vi "qnet_mechkit_decoder.vi"(1 "Reload Value":i16, 2 "Reset":bool, 3 "Z":bool, 4 "B":bool, 5 "A":bool, 6 "Enable Index":bool) -> (0 "16 bit Position":i16)   [LabVIEW 2017]
doc: "This contains a quadrature decoder with basic index support. When the index is enabled, the counter is reset to a specified value when the index pulse goes high or to zero if the reset button has been clicked."
uses:
  <vilib>/Simulation/Implementation/Shared/SIMSCR Execution Mode.ctl
  <vilib>/Simulation/Scripting/Companion Diagram/SimConfigNode/SimParams.ctl
  <vilib>/Simulation/Scripting/Companion Diagram/SimConfigNode/_simSolvers.ctl
  <vilib>/Simulation/Param Hierarchy/Typedefs/SIMPH Param Control Actions.ctl
  <vilib>/Simulation/Implementation/Shared/NILVSim_ParamChanged.vi
  <vilib>/Simulation/Implementation/Shared/NILVSIM_BeginStep.vi
  <vilib>/Simulation/Utility/Implementation/NILVSim Memory.llb/NILVSim Memory (core).vi
  <vilib>/Simulation/Implementation/Shared/NILVSim_Manager.vi
  <vilib>/Utility/error.llb/Clear Errors.vi
  <vilib>/Simulation/Implementation/Shared/NILVSim_FinalizeModel.vi
  <vilib>/Simulation/Implementation/Shared/SIM Unbundle Sim Info.vi
  <vilib>/Simulation/Implementation/Shared/SIMSH Read Queue.vi
  <vilib>/Simulation/Implementation/Shared/NILVSim_Initialize.vi
  <vilib>/Simulation/Utility/Implementation/NILVSim Get Time and IsAcceptedStep.vi
  <vilib>/Simulation/Implementation/Shared/NILVSim_GetModelError.vi
  <vilib>/Simulation/Implementation/Shared/SIM SimErrorHandler.vi
  <vilib>/Simulation/Implementation/Shared/SIM Bundle Sim Info.vi
  <vilib>/Simulation/Scripting/Companion Diagram/SimConfigNode/SimDog.xnode
  <vilib>/Simulation/Implementation/XNodeFramework/SimXNode/SimX.xnode
  <vilib>/Simulation/Implementation/Shared/NI_SIM_Implementation.lvlib
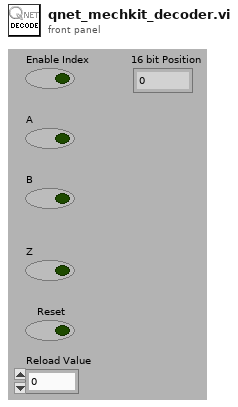
[diagram p1: front panel]
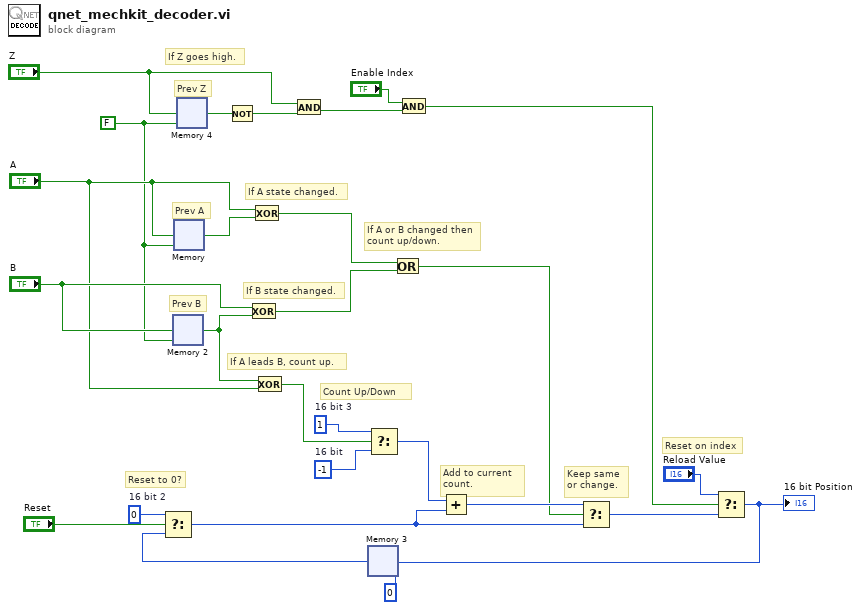
[diagram p0: block diagram]
diagram:
  w1 = FALSE ("initial value 2")
  w16 = i16 -1  # 16 bit
  w15 = i16 1  # 16 bit 3
  w11 = i16 0  # 16 bit 2
  # "Prev Z"
  # "If Z goes high."
  # "Add to current \ncount."
  # "Prev B"
  # "Prev A"
  # "Reset to 0?"
  # "Reset on index"
  # "Count Up/Down"
  # "Keep same \nor change."
  # "If A leads B, count up."
  # "If A state changed."
  # "If B state changed."
  # "If A or B changed then count up/down."
  n1 = xnode ("Memory 2")("input"="B", "initial value"=w1) -> ("output"=w20:bool)  [unwired: 4 in]
  n2 = xnode ("Memory")("input"="A", "initial value"=w1) -> ("output"=w19:bool)  [unwired: 4 in]
  n3 = xnode ("Memory 4")("input"="Z", "initial value"=w1) -> ("output"=w4:bool)  [unwired: 4 in]
  n4 = Not(x=w4) -> (.not. x?=w5:bool)
  n5 = Exclusive Or ("Exclusive Or 2")(1:w20, 2:"B") -> (0:w9:bool)
  n6 = Exclusive Or(1:w19, 2:"A") -> (0:w18:bool)
  n7 = Exclusive Or ("Exclusive Or 3")(1:"A", 2:w20) -> (0:w8:bool)
  n8 = And ("And 2")(x="Z", y=w5) -> (x .and. y?=w3:bool)
  n9 = Select ("Select 3")(t=w15, s=w8, f=w16) -> (s? t:f=w14:i16)
  n10 = Or(x=w18, y=w9) -> (x .or. y?=w7:bool)
  n11 = And(x="Enable Index", y=w3) -> (x .and. y?=w25:bool)
  n12 = Select ("Select 2")(t=w11, s="Reset", f=w21) -> (s? t:f=w12:i16)
  n13 = Add(x=w14, y=w12) -> (x+y=w10:i16)
  n14 = Select(t=w10, s=w7, f=w12) -> (s? t:f=w17:i16)
  n15 = Select ("Select 4")(t="Reload Value", s=w25, f=w17) -> (s? t:f=w27:i16)
  "16 bit Position" <- w27
  n16 = xnode ("Memory 3")("input"=w27, "initial value"=i16 0) -> ("output"=w21:i16)  [unwired: 4 in]
